vi "Analyze Data.vi"(8 "error in":errorcluster, 11 "cCRDS in":refnum<class "cCRDS.lvclass">) -> (0 "error out":errorcluster, 3 "cCRDS out":refnum<class "cCRDS.lvclass">)   [LabVIEW 2015, in "cCRDS.lvclass"]
doc: "Analyze Data takes the stored ringdown data (1000 shots per cell) and:\n1) Calculates the ringdown decay constant tau\n2) Averages tau0 data as necessary\n3) Corrects the tau data for Rayleigh scattering\n4) Stores a 1-D array of taus returned on a 1 kHz basis (8k taus) if a jump drive (U:) is connected\n5) Flattens the data into a string and stuffs the string into the <b>data</b> shared variable for display on the UI.\n\nThis VI will not be called if the data is not \"good\" (that is, if an error was thrown in the <B>Get Data</B> routine. If an error is thrown while the data is being retrieved, then the data will not be sent to the UI."
uses:
  cCRDS.lvclass
  Reusable/CRDS/Data/Cell/CRDS Cell Data.lvclass/CRDS Cell Data.ctl
  Reusable/CRDS/Data/Cell/Read extParam.vi
  Reusable/CRDS/Data/Cell/Write extParam.vi
  Reusable/CRDS/Main/Read Data.vi
  Reusable/CRDS/Data/Main/Read CellData.vi
  Reusable/CRDS/Data/Main/Write CellData.vi
  Reusable/CRDS/Main/CRDS.lvclass
  Reusable/CRDS/Data/Main/CRDS Data.lvclass
  Reusable/CRDS/Data/Cell/CRDS Cell Data.lvclass
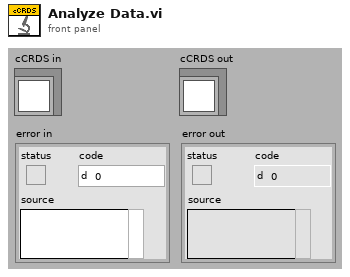
[diagram p1: front panel]
types:
  T1 = typedef "extparam.ctl" = cluster{"Tau":sgl, "Tau0cor":sgl, "ext":sgl, "extCorr":sgl, "stdevTau":sgl, "eTau":sgl, "taucorr":sgl, "Tau0":sgl, "max":sgl}
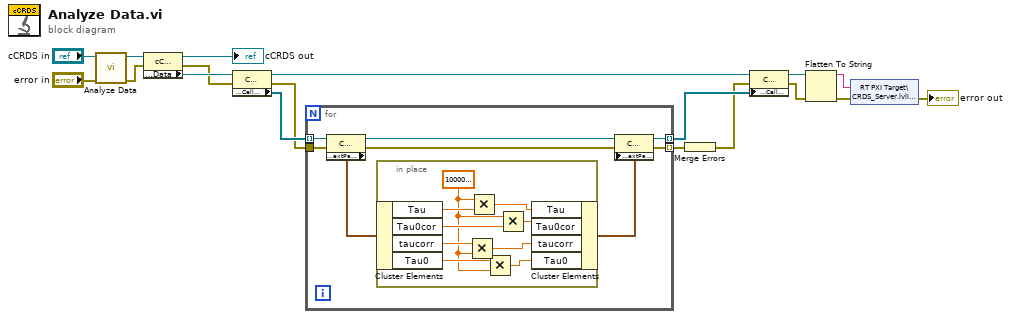
[diagram p0: block diagram]
diagram:
  n1 = call-parent "Analyze Data.vi"("error in"="error in", "CRDS in"="cCRDS in") -> ("error out"=w15:errorcluster, "CRDS out"=w16:refnum<class "cCRDS.lvclass">)  [unwired: 8 in]
  n2 = property class="cCRDS"(reference=w16, error in=w15) -> (reference out=→"cCRDS out":refnum<class "cCRDS.lvclass">, error out=w4:errorcluster, "Data Access:Data"=w10:refnum<class "CRDS Data.lvclass">)
  n3 = property class="CRDS"(reference=w10, error in=w4) -> (reference out=w7:refnum<class "CRDS Data.lvclass">, error out=w3:errorcluster, "Data Access:Cell Data"=w9:refnum<class "CRDS Cell Data.lvclass">[])
  n4 = for {
    tunnel: w9 -> [w26] mode=indexing
    tunnel: [w24] -> w8 mode=indexing
    tunnel: [w20] -> w5 mode=indexing
    tunnel: w3 -> [w19]
    n5 = property class="CRDS Cell"(reference=w26, error in=w19) -> (reference out=w25:refnum<class "CRDS Cell Data.lvclass">, error out=w21:errorcluster, "Data Access:extParam"=w23:T1)
    n6 = in-place {
      w27 = sgl 1000000.0 ("x")
      n7 = in-place-cluster #1(w23) -> ("Tau"=w35:sgl, "Tau0cor"=w33:sgl, "taucorr"=w31:sgl, "Tau0"=w29:sgl)
      n8 = Multiply(x=w31, y=w27) -> (x*y=w30:sgl)
      n9 = Multiply(x=w27, y=w35) -> (x*y=w34:sgl)
      n10 = Multiply(x=w29, y=w27) -> (x*y=w28:sgl)
      n11 = Multiply(x=w27, y=w33) -> (x*y=w32:sgl)
      n12 = in-place-cluster #1("Tau"=w34, "Tau0cor"=w32, "taucorr"=w30, "Tau0"=w28) -> (w22:T1)
    }
    n13 = property class="CRDS Cell"(reference=w25, error in=w21, "Data Access:extParam"=w22) -> (reference out=w24:refnum<class "CRDS Cell Data.lvclass">, error out=w20:errorcluster)
  }
  n14 = Merge Errors(w5) -> (w2:errorcluster)
  n15 = property class="CRDS"(reference=w7, error in=w2, "Data Access:Cell Data"=w8) -> (reference out=w6:refnum<class "CRDS Data.lvclass">, error out=w1:errorcluster)
  n16 = Flatten To String(anything=w6, error in (no error)=w1) -> (data string=w12:string, error out=w14:errorcluster)  [unwired: 2 in, 1 out]
  n17 = shared-variable "RT PXI Target\\CRDS_Server.lvlib\\data"(w12, error in=w14) -> (error out=→"error out":errorcluster)
